vi "CLIENT_check_if_error_already_displayed.vi"(8 "error_in":errorcluster, 10 "thread_in":T1, 11 "displayed_errors":i32[][](array[numeric])) -> (1 "error_code":i32, 2 "thread_out":T1, 3 "already_displayed?":bool)   [LabVIEW 2019]
uses:
  MAIN/thread_name.ctl
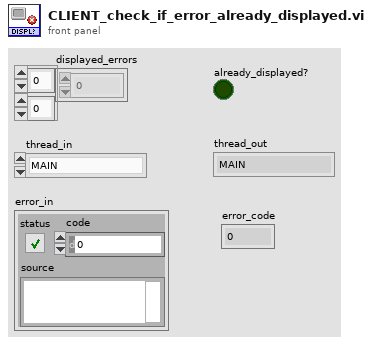
[diagram p1: front panel]
types:
  T1 = typedef "thread_name.ctl" = enum16{"MAIN"}
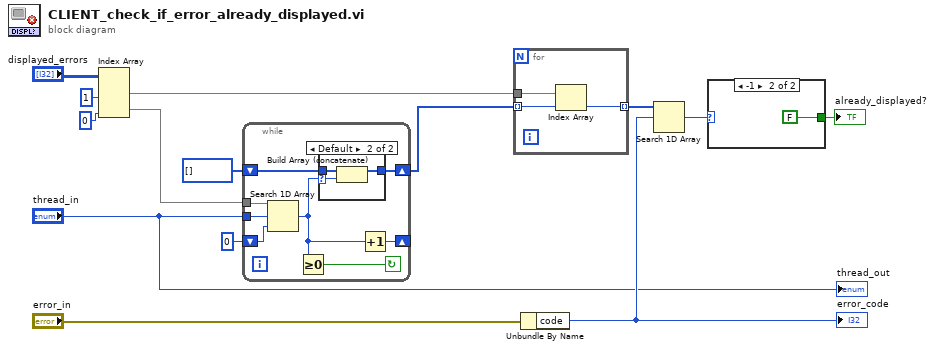
[diagram p0: block diagram]
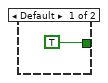
[diagram p2: hidden frame]
diagram:
  n1 = Index Array(array="displayed_errors", index (col) #1=1 ("disabled index (col)"), index (col) #2=0 ("index (col)")) -> (element #1=w1:i32[], element #2=w2:i32[])  [unwired: 2 in]
  n2 = while {
    shift-right: [w15] -> _
    shift-left: 0 -> [w22]
    shift-right: [w19] -> w7
    shift-left: i32[] [] ("Initial Elements") -> [w20]
    tunnel: w2 -> [w21]
    tunnel: "thread_in" -> [w18]
    stop <- w16 continue-if-true
    n3 = Search 1D Array(1D array=w21, element=w18, start index (0)=w22) -> (index of element=w17:i32)
    n4 = Greater Or Equal To 0?(x=w17) -> (x >= 0?=w16:bool)
    n5 = case shown="Default" w17 {
      selector: w17 -> [_ w26]
      tunnel: w20 -> [w23 w25]
      tunnel: [w23 w24] -> w19
      frame -1 {
      }
      frame Default {
        n6 = Build Array (concatenate)(w25, w26) -> (w24:i32[])
      }
    }
    n7 = Increment(x=w17) -> (x+1=w15:i32)
  }
  n8 = for {
    tunnel: w7 -> [w29] mode=indexing
    tunnel: w1 -> [w28]
    tunnel: [w27] -> w8 mode=indexing
    n9 = Index Array(array=w28, index=w29) -> (element=w27:i32)
  }
  n10 = Unbundle By Name("error_in") -> ("code"=w12:i32)
  "error_code" <- w12
  n11 = Search 1D Array(1D array=w8, element=w12) -> (index of element=w6:i32)  [unwired: 1 in]
  n12 = case shown="-1" w6 {
    tunnel: [TRUE FALSE] -> w5
    frame Default {
    }
    frame -1 {
    }
  }
  "already_displayed?" <- w5
  "thread_out" <- "thread_in"
